vi "AH2500_read_parameters_visa.vi"(0 "VISA-AH2500":refnum<visa-resource-name>, 3 "error in (no error)":errorcluster caption="Fehler (Eingang, kein Fehler)") -> (4 "VISA-AH2500 dub":refnum<visa-resource-name>, 5 "error out":errorcluster caption="Fehler (Ausgang)", 6 "AVerage":T2(ring)=enum."5", 7 "ALternate":enum16{"0", "1", "2", "3", "4", "5", "6", "7"}(ring)=enum."1", 8 "BIas":enum16{"Disabled", "100 MOhm", "1 MOhm"}(ring), 9 "V excitation 2":T1(ring))   [LabVIEW 2018]
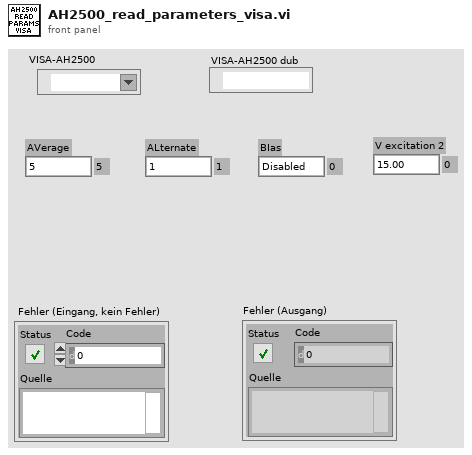
[diagram p1: front panel]
types:
  T1 = enum16{"15.00", "7.50", "3.75", "3.00", "1.50", "0.750", "0.375", "0.250", "0.125", "0.100", "0.050", "0.030", "0.015", "0.010", "0.0050", "0.0030", "0.0015", "0.0010", "0.0005"}
  T2 = enum16{"0", "1", "2", "3", "4", "5", "6", "7", "8", "9", "10", "11", "12", "13", "14", "15"}
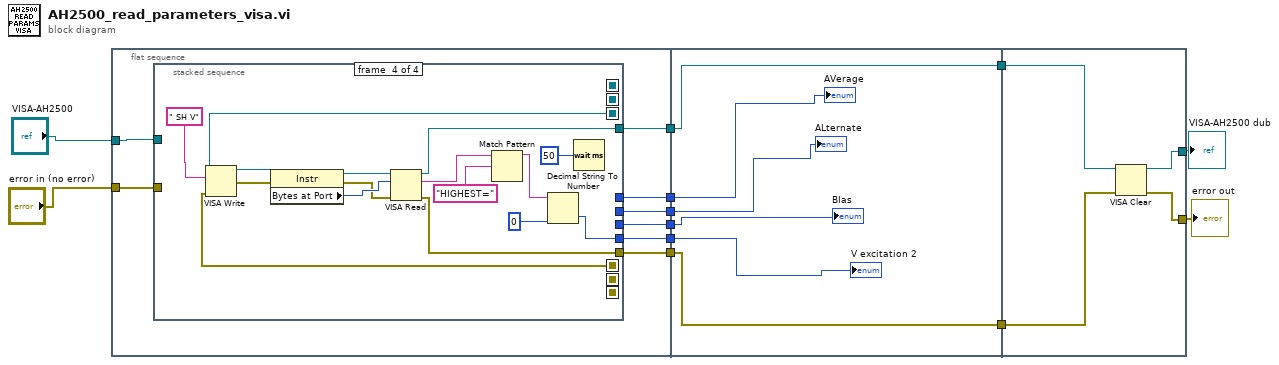
[diagram p0: block diagram]
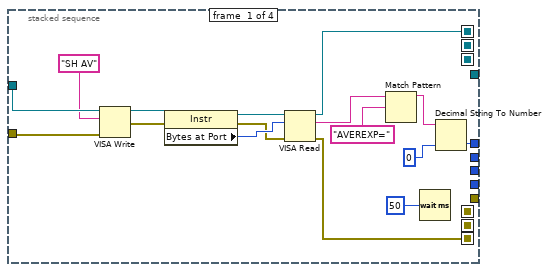
[diagram p2: hidden frame]
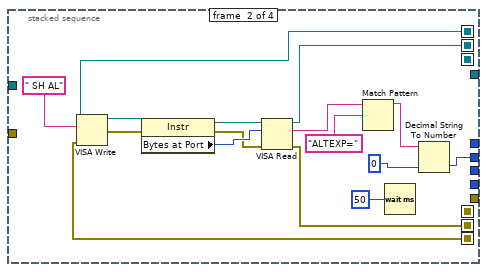
[diagram p3: hidden frame]
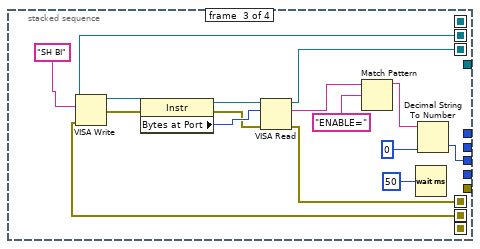
[diagram p4: hidden frame]
diagram:
  n1 = flat-sequence {
    tunnel: "error in (no error)" -> [w19]
    tunnel: "VISA-AH2500" -> [w20]
    tunnel: [w18] -> w6
    tunnel: [w17] -> w5
    tunnel: [w16] -> w4
    tunnel: [w15] -> w3
    tunnel: [w14] -> w2
    tunnel: [w13] -> w1
    tunnel: [w89] -> w8
    tunnel: [w90] -> w7
    tunnel: w6 -> [w88]
    tunnel: w5 -> [w87]
    tunnel: w4 -> [w85]
    tunnel: w3 -> [w86]
    tunnel: w2 -> [w90]
    tunnel: w1 -> [w89]
    tunnel: [w92] -> w9
    tunnel: [w91] -> w10
    tunnel: w8 -> [w94]
    tunnel: w7 -> [w93]
    frame #0 {
      n2 = stacked-sequence {
        seq-local: [w31 _ _ _] -> [_ w43 _ _]
        seq-local: [w30 _ _ _] -> [_ w42 _ _]
        seq-local: [_ w41 _ _] -> [_ _ w58 _]
        seq-local: [_ w40 _ _] -> [_ _ w57 _]
        seq-local: [_ _ w56 _] -> [_ _ _ w75]
        seq-local: [_ _ w55 _] -> [_ _ _ w74]
        tunnel: w20 -> [w29 _ _ _]
        tunnel: w19 -> [w27 _ _ _]
        tunnel: [w23 _ _ _] -> w18
        tunnel: [_ w39 _ _] -> w17
        tunnel: [_ _ w59 _] -> w16
        tunnel: [_ _ _ w73] -> w15
        tunnel: [_ _ _ w71] -> w14
        tunnel: [_ _ _ w70] -> w13
        frame #0 {
          n3 = VISA Write(VISA resource name=w29, write buffer="SH AV", error in (no error)=w27) -> (VISA resource name out=w35:refnum<visa-resource-name>, error out=w36:errorcluster)  [unwired: 1 out]
          n4 = property class="Instr"(reference=w35, error in=w36) -> (reference out=w34:refnum<visa-resource-name>, error out=w32:errorcluster, "Bytes at Port"=w33:u32)
          n5 = VISA Read(VISA resource name=w34, byte count=w33, error in (no error)=w32) -> (VISA resource name out=w31:refnum<visa-resource-name>, read buffer=w25:string, error out=w30:errorcluster)  [unwired: 1 out]
          n6 = Match Pattern(string=w25, regular expression="AVEREXP=") -> (before substring=w24:string)  [unwired: 1 in, 3 out]
          n7 = Wait (ms)(milliseconds to wait=50) -> ()  [unwired: 1 out]
          n8 = Decimal String To Number(string=w24, default (0L)=0) -> (number=w23:i32)  [unwired: 1 in, 1 out]
        }
        frame #1 {
          n9 = VISA Write(VISA resource name=w43, write buffer=" SH AL", error in (no error)=w42) -> (VISA resource name out=w51:refnum<visa-resource-name>, error out=w52:errorcluster)  [unwired: 1 out]
          n10 = property class="Instr"(reference=w51, error in=w52) -> (reference out=w50:refnum<visa-resource-name>, error out=w48:errorcluster, "Bytes at Port"=w49:u32)
          n11 = VISA Read(VISA resource name=w50, byte count=w49, error in (no error)=w48) -> (VISA resource name out=w41:refnum<visa-resource-name>, read buffer=w45:string, error out=w40:errorcluster)  [unwired: 1 out]
          n12 = Match Pattern(string=w45, regular expression="ALTEXP=") -> (before substring=w44:string)  [unwired: 1 in, 3 out]
          n13 = Wait (ms)(milliseconds to wait=50) -> ()  [unwired: 1 out]
          n14 = Decimal String To Number(string=w44, default (0L)=0) -> (number=w39:i32)  [unwired: 1 in, 1 out]
        }
        frame #2 {
          n15 = VISA Write(VISA resource name=w58, write buffer="SH BI", error in (no error)=w57) -> (VISA resource name out=w67:refnum<visa-resource-name>, error out=w68:errorcluster)  [unwired: 1 out]
          n16 = property class="Instr"(reference=w67, error in=w68) -> (reference out=w66:refnum<visa-resource-name>, error out=w64:errorcluster, "Bytes at Port"=w65:u32)
          n17 = VISA Read(VISA resource name=w66, byte count=w65, error in (no error)=w64) -> (VISA resource name out=w56:refnum<visa-resource-name>, read buffer=w61:string, error out=w55:errorcluster)  [unwired: 1 out]
          n18 = Match Pattern(string=w61, regular expression="ENABLE=") -> (before substring=w60:string)  [unwired: 1 in, 3 out]
          n19 = Wait (ms)(milliseconds to wait=50) -> ()  [unwired: 1 out]
          n20 = Decimal String To Number(string=w60, default (0L)=0) -> (number=w59:i32)  [unwired: 1 in, 1 out]
        }
        frame #3 {
          n21 = VISA Write(VISA resource name=w75, write buffer=" SH V", error in (no error)=w74) -> (VISA resource name out=w83:refnum<visa-resource-name>, error out=w84:errorcluster)  [unwired: 1 out]
          n22 = property class="Instr"(reference=w83, error in=w84) -> (reference out=w82:refnum<visa-resource-name>, error out=w80:errorcluster, "Bytes at Port"=w81:u32)
          n23 = VISA Read(VISA resource name=w82, byte count=w81, error in (no error)=w80) -> (VISA resource name out=w71:refnum<visa-resource-name>, read buffer=w77:string, error out=w70:errorcluster)  [unwired: 1 out]
          n24 = Match Pattern(string=w77, regular expression="HIGHEST=") -> (before substring=w76:string)  [unwired: 1 in, 3 out]
          n25 = Decimal String To Number(string=w76, default (0L)=0) -> (number=w73:i32)  [unwired: 1 in, 1 out]
          n26 = Wait (ms)(milliseconds to wait=50) -> ()  [unwired: 1 out]
        }
      }
    }
    frame #1 {
      "AVerage" <- w88
      "ALternate" <- w87
      "BIas" <- w85
      "V excitation 2" <- w86
    }
    frame #2 {
      n27 = VISA Clear(VISA resource name=w93, error in (no error)=w94) -> (VISA resource name out=w91:refnum<visa-resource-name>, error out=w92:errorcluster)
    }
  }
  "VISA-AH2500 dub" <- w10
  "error out" <- w9
